vi "Close MeasurementLink Session.vi"(8 "error in":errorcluster, 9 "close session behavior":T1, 10 "session in":variant, 11 "instrument in":refnum<class "Instrument.lvclass">) -> (0 "error out":errorcluster)   [LabVIEW 2020, in "MeasurementLink niFGEN.lvlib" / "Instrument.lvclass"]
uses:
  Instrument.lvclass
  MeasurementLink Instrument/IInstrument/Close Session Behavior.ctl
  Instrument.lvclass/Instrument.ctl
  MeasurementLink Measurement Server/Helpers/Error Strings Global Internal.vi
  MeasurementLink Instrument/IInstrument/IInstrument.lvclass
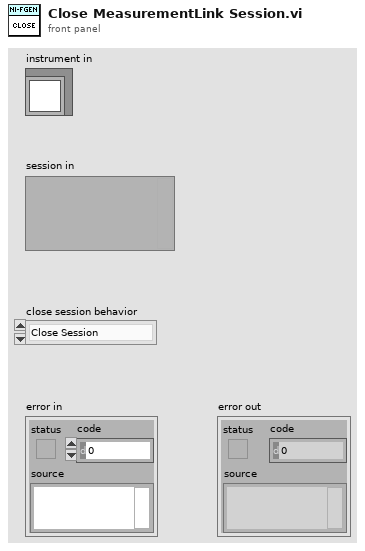
[diagram p1: front panel]
types:
  T1 = typedef "MeasurementLink Instrument.lvlib/IInstrument.lvclass/Close Session Behavior.ctl" = enum16{"Close Session", "Detach Session"}
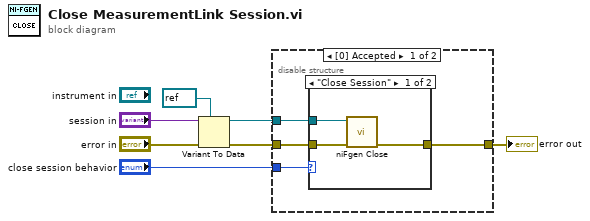
[diagram p0: block diagram]
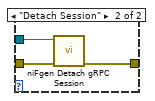
[diagram p2: hidden frame]
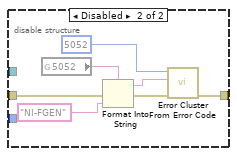
[diagram p3: hidden frame]
diagram:
  n1 = Variant To Data(error in="error in", type=refnum<k15> refnum ("Instrument Handle"), Variant="session in") -> (data=w1:refnum<k15>, error out=w2:errorcluster)
  n2 = disable-structure shown="[0] Accepted" {
    disable-tunnel: "close session behavior" -> [w8 _]
    disable-tunnel: w2 -> [w9 w18]
    disable-tunnel: w1 -> [w10 _]
    disable-tunnel: [w11 w24] -> w4
    frame Enabled {
      n3 = case shown="\"Close Session\"" w8 {
        tunnel: w9 -> [w14 w17]
        tunnel: w10 -> [w12 w16]
        tunnel: [w13 w15] -> w11
        frame "Close Session" {
          n4 = call <instrlib>:"niFgen Close.vi"("error in (no error)"=w14, "Instrument Handle"=w12) -> ("error out"=w13:errorcluster)  [unwired: 9 in]
        }
        frame "Detach Session" {
          n5 = call <instrlib>:"niFgen Detach gRPC Session.vi"("error in (no error)"=w17, "Instrument Handle"=w16) -> ("error out"=w15:errorcluster)  [unwired: 9 in]
        }
      }
    }
    frame Disabled {
      n6 = global read "Error Strings Global Internal.vi" "5052"() -> (w22:string)
      n7 = Format Into String(format string=w22, error in=w18, "NI-FGEN") -> (resulting string=w19:string, error out=w20:errorcluster)  [unwired: 1 in]
      n8 = call <vilib>:"Error Cluster From Error Code.vi"("error in (no error)"=w20, "error message (\"\")"=w19, "error code (0)"=5052) -> ("error out"=w24:errorcluster)  [unwired: 6 in]
    }
  }
  "error out" <- w4
